vi "Configure Modulation (LF Output).vi"(0 "VISA resource name":refnum<visa-resource-name>, 1 "Enable Low Frequency Output (F: Disable)":bool, 2 "Monitor Source (0: Function 1)":i32(ring) items=["Function 1", "Function 2", "Sweep", "Dual"], 5 "Low Frequency Output Amplitude (0 VP)":dbl, 7 "Load Impedance (50: 50 Ohm)":i32(ring)=50 items=["50 Ohm"=50, "1000000 Ohm"=1000000], 9 "DC Offset (0 V)":dbl, 11 "error in (no error)":errorcluster, 12 "Low Frequency Source (0: Monitor)":i32(ring) items=["Monitor", "Function 1", "Function 2", "Sweep", "Dual", "Noise 1", "Noise 2", "DC"]) -> (4 "VISA resource name out":refnum<visa-resource-name>, 15 "error out":errorcluster)   [LabVIEW 2014, in "Agilent PSG MXG Series.lvlib"]
doc: "Configures the low frequency output for MXG-B, EXG-B Series.\n\n<B>Notes:</B>\n(1) This VI is valid only in N5162A, N5182A, N5172B, N5182B that install <B>Option UNT</B>."
uses:
  Agilent PSG MXG Series.lvlib
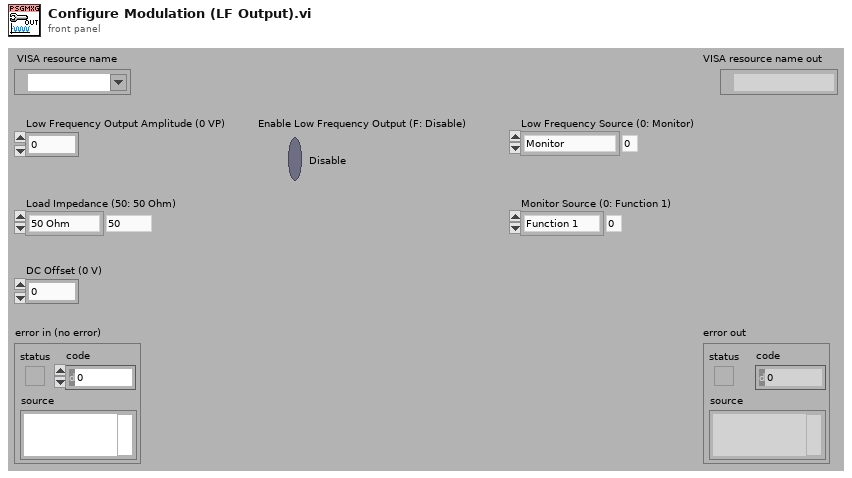
[diagram p1: front panel]
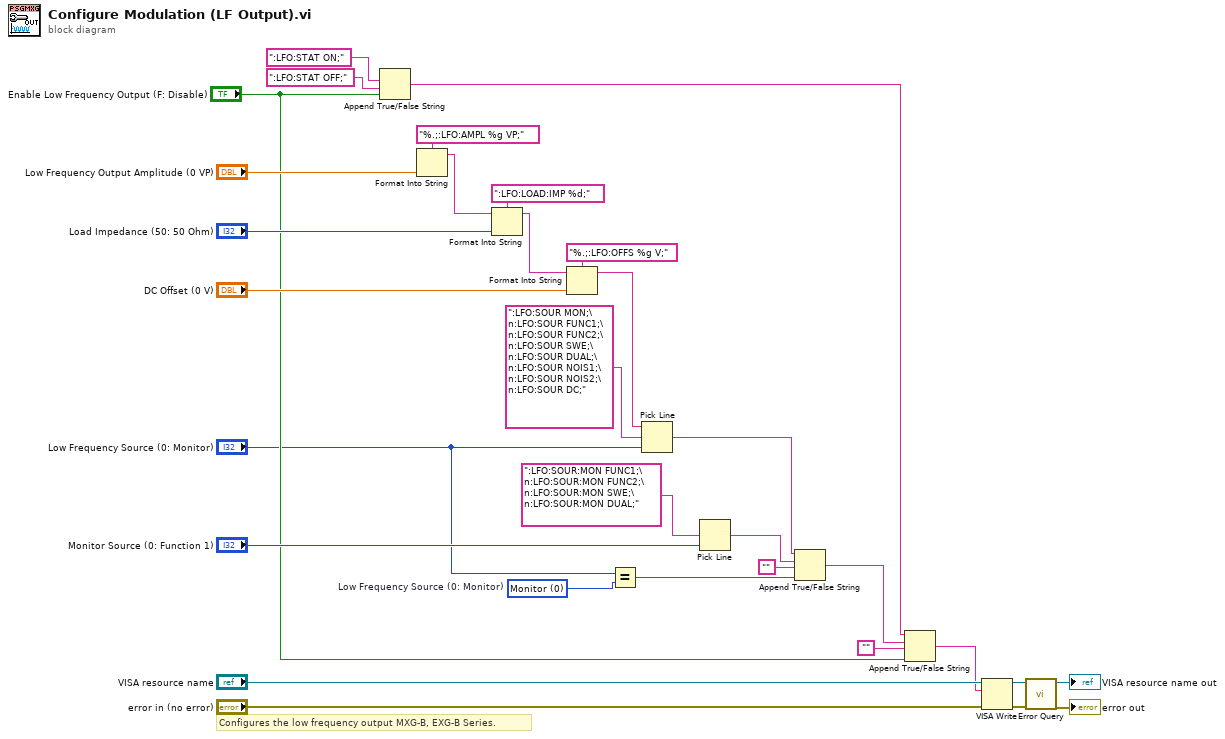
[diagram p0: block diagram]
diagram:
  w3 = 0 items=["Monitor", "Function 1", "Function 2", "Sweep", "Dual", "Noise 1", "Noise 2", "DC"]  # Low Frequency Source (0: Monitor)
  # "Configures the low frequency output MXG-B, EXG-B Series."
  n1 = Append True/False String(1:"Enable Low Frequency Output (F: Disable)", 2:":LFO:STAT OFF;", 3:":LFO:STAT ON;") -> (0:w11:string)  [unwired: 1 out]
  n2 = Format Into String(format string="%.;:LFO:AMPL %g VP;", "Low Frequency Output Amplitude (0 VP)") -> (resulting string=w29:string)  [unwired: 2 in, 1 out]
  n3 = Format Into String(format string=":LFO:LOAD:IMP %d;", initial string=w29, "Load Impedance (50: 50 Ohm)") -> (resulting string=w26:string)  [unwired: 1 in, 1 out]
  n4 = Format Into String(format string="%.;:LFO:OFFS %g V;", initial string=w26, "DC Offset (0 V)") -> (resulting string=w22:string)  [unwired: 1 in, 1 out]
  n5 = Equal?(x="Low Frequency Source (0: Monitor)", y=w3) -> (x = y?=w2:bool)
  n6 = Pick Line(string ("")=w22, multi-line string=":LFO:SOUR MON;\n:LFO:SOUR FUNC1;\n:LFO:SOUR FUNC2;\n:LFO:SOUR SWE;\n:LFO:SOUR DUAL;\n:LFO:SOUR NOIS1;\n:LFO:SOUR NOIS2;\n:LFO:SOUR DC;", line index="Low Frequency Source (0: Monitor)") -> (output string=w5:string)
  n7 = Pick Line(multi-line string=":LFO:SOUR:MON FUNC1;\n:LFO:SOUR:MON FUNC2;\n:LFO:SOUR:MON SWE;\n:LFO:SOUR:MON DUAL;", line index="Monitor Source (0: Function 1)") -> (output string=w6:string)  [unwired: 1 out]
  n8 = Append True/False String(1:w2, 2:"", 3:w6, 4:w5) -> (0:w1:string)
  n9 = Append True/False String(1:"Enable Low Frequency Output (F: Disable)", 2:"", 3:w1, 4:w11) -> (0:w8:string)
  n10 = VISA Write(VISA resource name="VISA resource name", write buffer=w8, error in (no error)="error in (no error)") -> (VISA resource name out=w16:refnum<visa-resource-name>, error out=w15:errorcluster)  [unwired: 1 out]
  n11 = call "Error Query.vi"("error in (no error)"=w15, "VISA resource name"=w16) -> ("error out"=→"error out":errorcluster, "VISA resource name out"=→"VISA resource name out":refnum<visa-resource-name>)  [unwired: 8 out]
